vi "Check if subpanel open.vi"() -> (0 "Proceed / Subpanel is not open":bool)   [LabVIEW 2013]
uses:
  Typedefs/Set Main VI cursor.ctl
  Typedefs/Subpanel close request.ctl
  Global Variables/General Globals.vi
  Global Variables/gl_Queues.vi
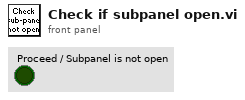
[diagram p1: front panel]
types:
  T1 = typedef "Set Main VI cursor.ctl" = enum16{"Release busy cursor", "Set busy cursor"}
  T2 = typedef "Subpanel close request.ctl" = enum16{"Request subpanel close", "Just check subpanel is closed"}
  T3 = typedef "All Message Queues.ctl" = cluster{"UI queue":refnum<queue>, "Acq. queue":refnum<queue>, "Logging queue":refnum<queue>}
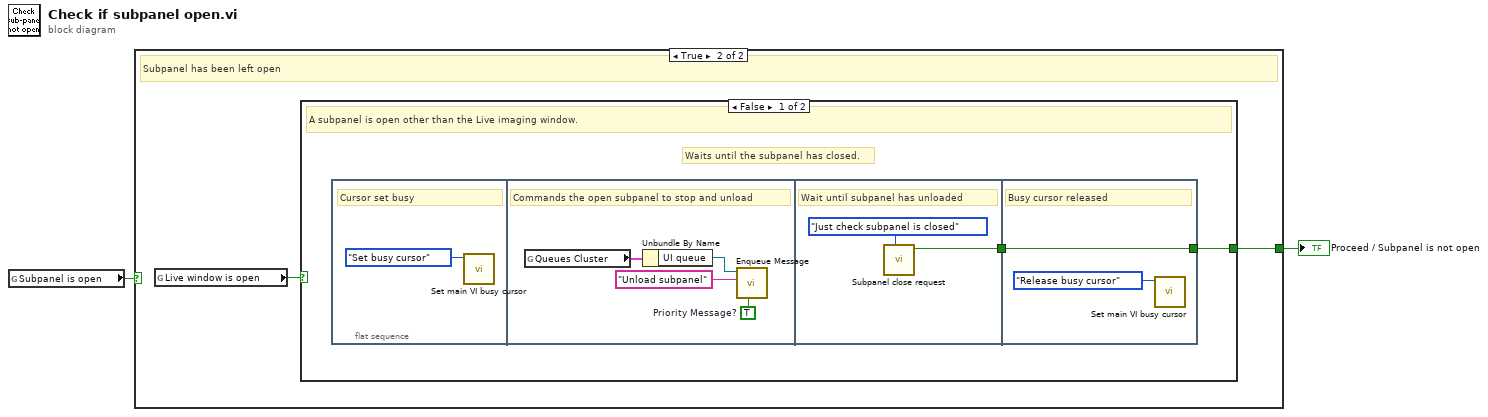
[diagram p0: block diagram]
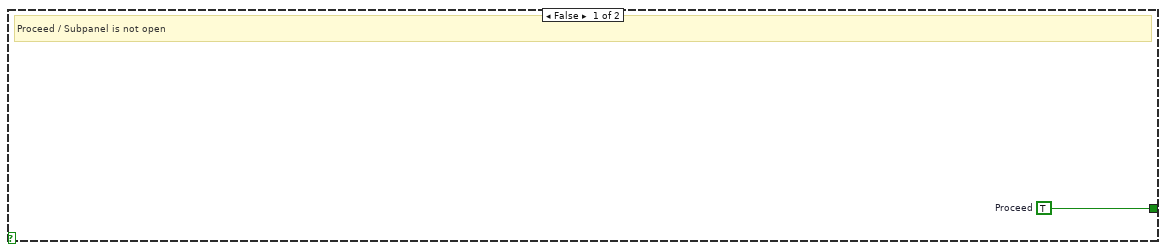
[diagram p2: hidden frame]
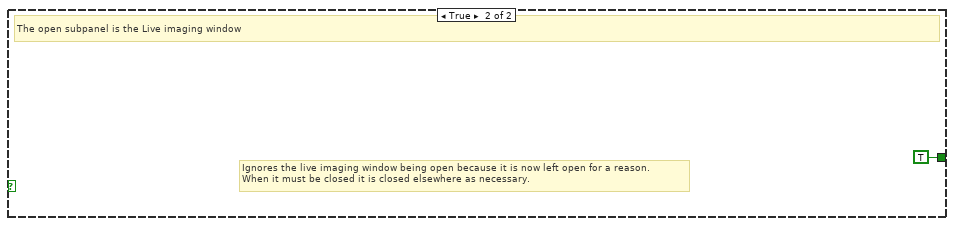
[diagram p3: hidden frame]
diagram:
  n1 = global read "General Globals.vi" "Subpanel is open"() -> (w2:bool)
  n2 = case shown="True" w2 {
    tunnel: [w3 w5] -> w1
    frame False {
      w3 = TRUE  # Proceed
      # "Proceed / Subpanel is not open"
    }
    frame True {
      # "Subpanel has been left open"
      n3 = global read "General Globals.vi" "Live window is open"() -> (w4:bool)
      n4 = case shown="False" w4 {
        tunnel: [w6 TRUE ("Subpanel is closed / Proceed")] -> w5
        frame False {
          # "Waits until the subpanel has closed."
          # "A subpanel is open other than the Live imaging window."
          n5 = flat-sequence {
            tunnel: [w14] -> w7
            tunnel: [w15] -> w6
            tunnel: w7 -> [w15]
            frame #0 {
              # "Cursor set busy"
              n6 = call "Set main VI busy cursor.vi"("Main VI's cursor"=Set_Main_VI_cursor."Set busy cursor") -> ()  [unwired: 10 in, 1 out]
            }
            frame #1 {
              w12 = TRUE  # Priority Message?
              # "Commands the open subpanel to stop and unload"
              n7 = global read "gl_Queues.vi" "Queues Cluster"() -> (w10:T3)
              n8 = Unbundle By Name(w10) -> ("UI queue"=w9:refnum<queue>)
              n9 = call "Enqueue Message.vi"("Priority Message? (F)"=w12, "Message"="Unload subpanel", "Queue"=w9) -> ()  [unwired: 7 in, 2 out]
            }
            frame #2 {
              # "Wait until subpanel has unloaded"
              n10 = call "Subpanel close request.vi"("Function"=Subpanel_close_request."Just check subpanel is closed") -> ("Subpanel is closed / Proceed"=w14:bool)  [unwired: 10 in]
            }
            frame #3 {
              # "Busy cursor released"
              n11 = call "Set main VI busy cursor.vi"("Main VI's cursor"=Set_Main_VI_cursor."Release busy cursor") -> ()  [unwired: 10 in, 1 out]
            }
          }
        }
        frame True {
          # "Ignores the live imaging window being open because it is now left open for a reason.\nWhen it must be closed it is closed elsewhere as necessary."
          # "The open subpanel is the Live imaging window"
        }
      }
    }
  }
  "Proceed / Subpanel is not open" <- w1
